vi "gaussian.vi"() -> ()   [LabVIEW 2015]
panel:
  out "Intensity Chart":dbl[][](graph)
  out "Waveform Chart":dbl[](graph)
  out "size(s)":i32
  in  "sigma":dbl(slide)=0.5 scale=-5.0..5.0
  in  "kernelSize":enum16{"3x3", "5x5", "7x7"}(ring)
  out "G":dbl[][](array[numeric])
  in  "dX":dbl=1.0 format="%#_13g"
  in  "sigma":dbl=0.8493
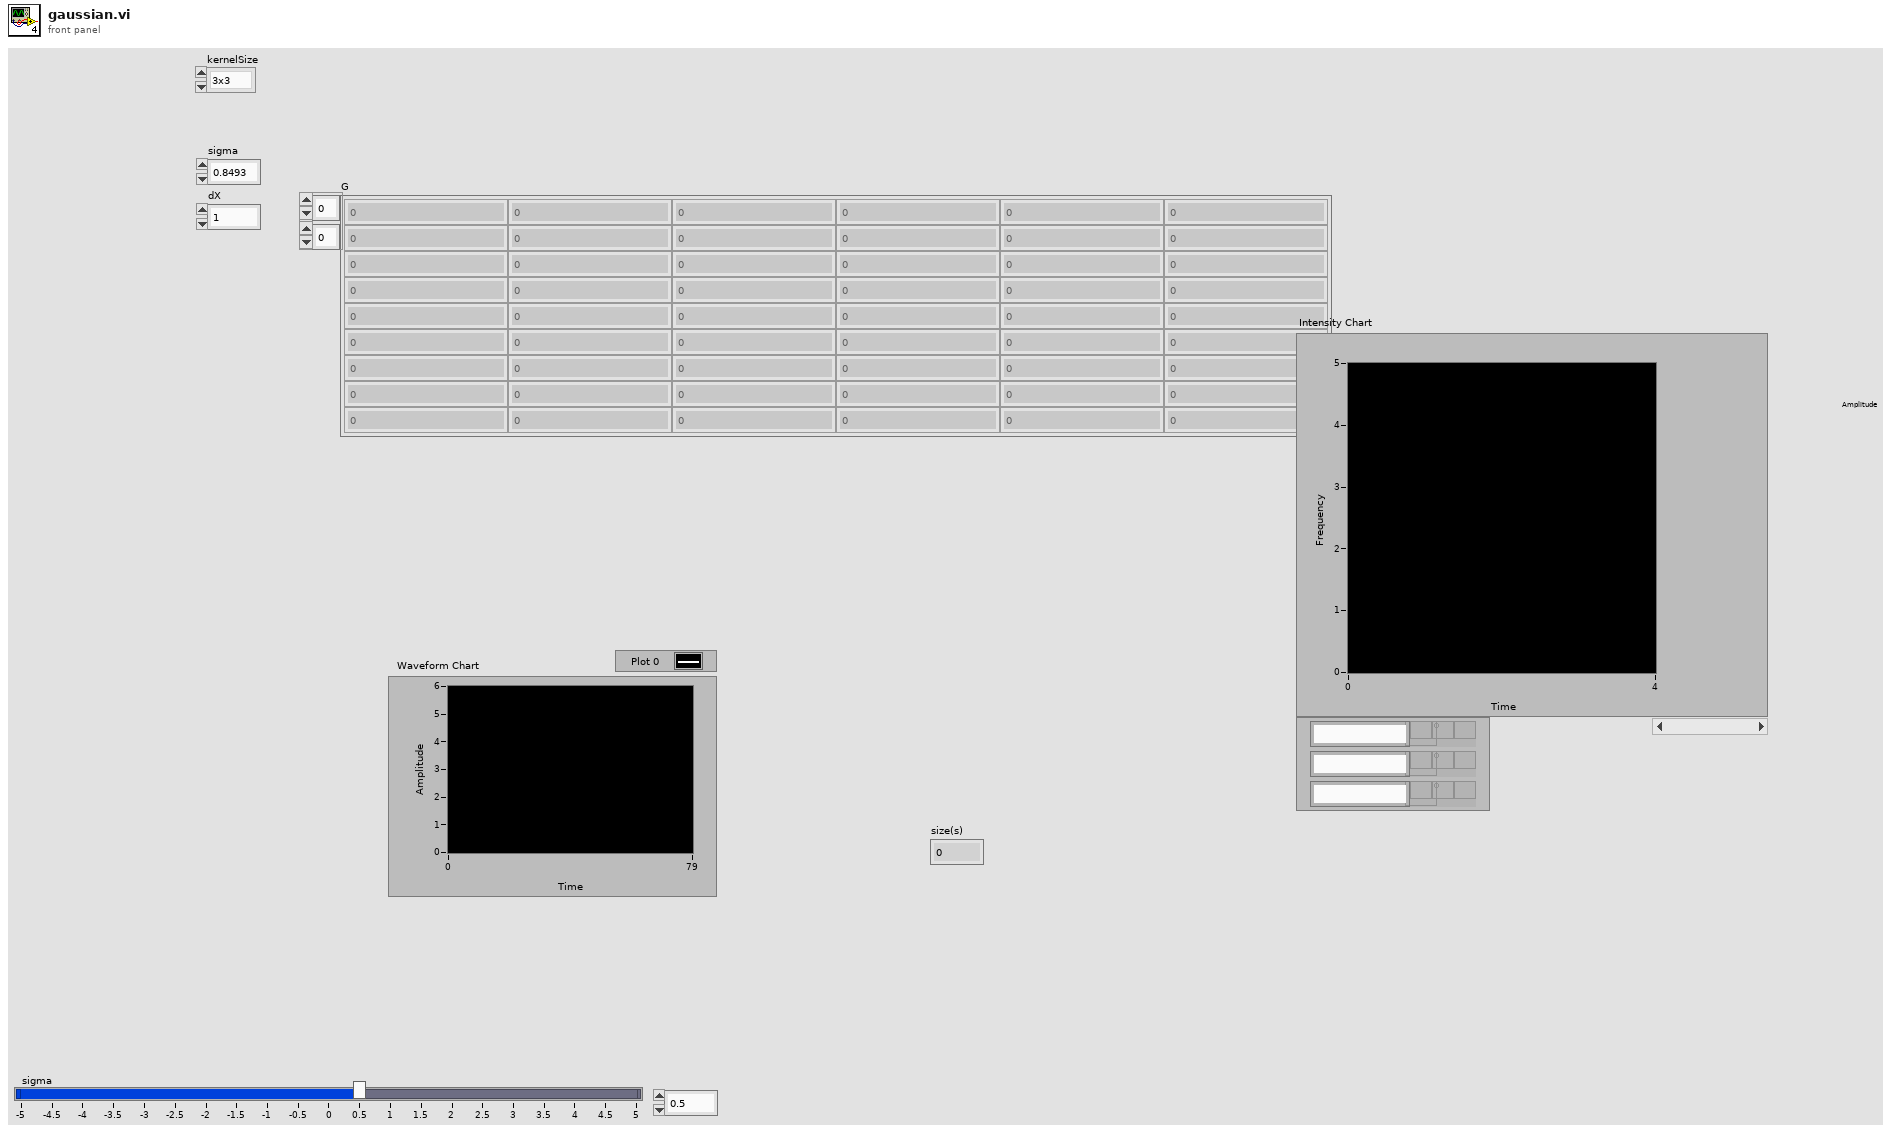
[diagram p1: front panel]
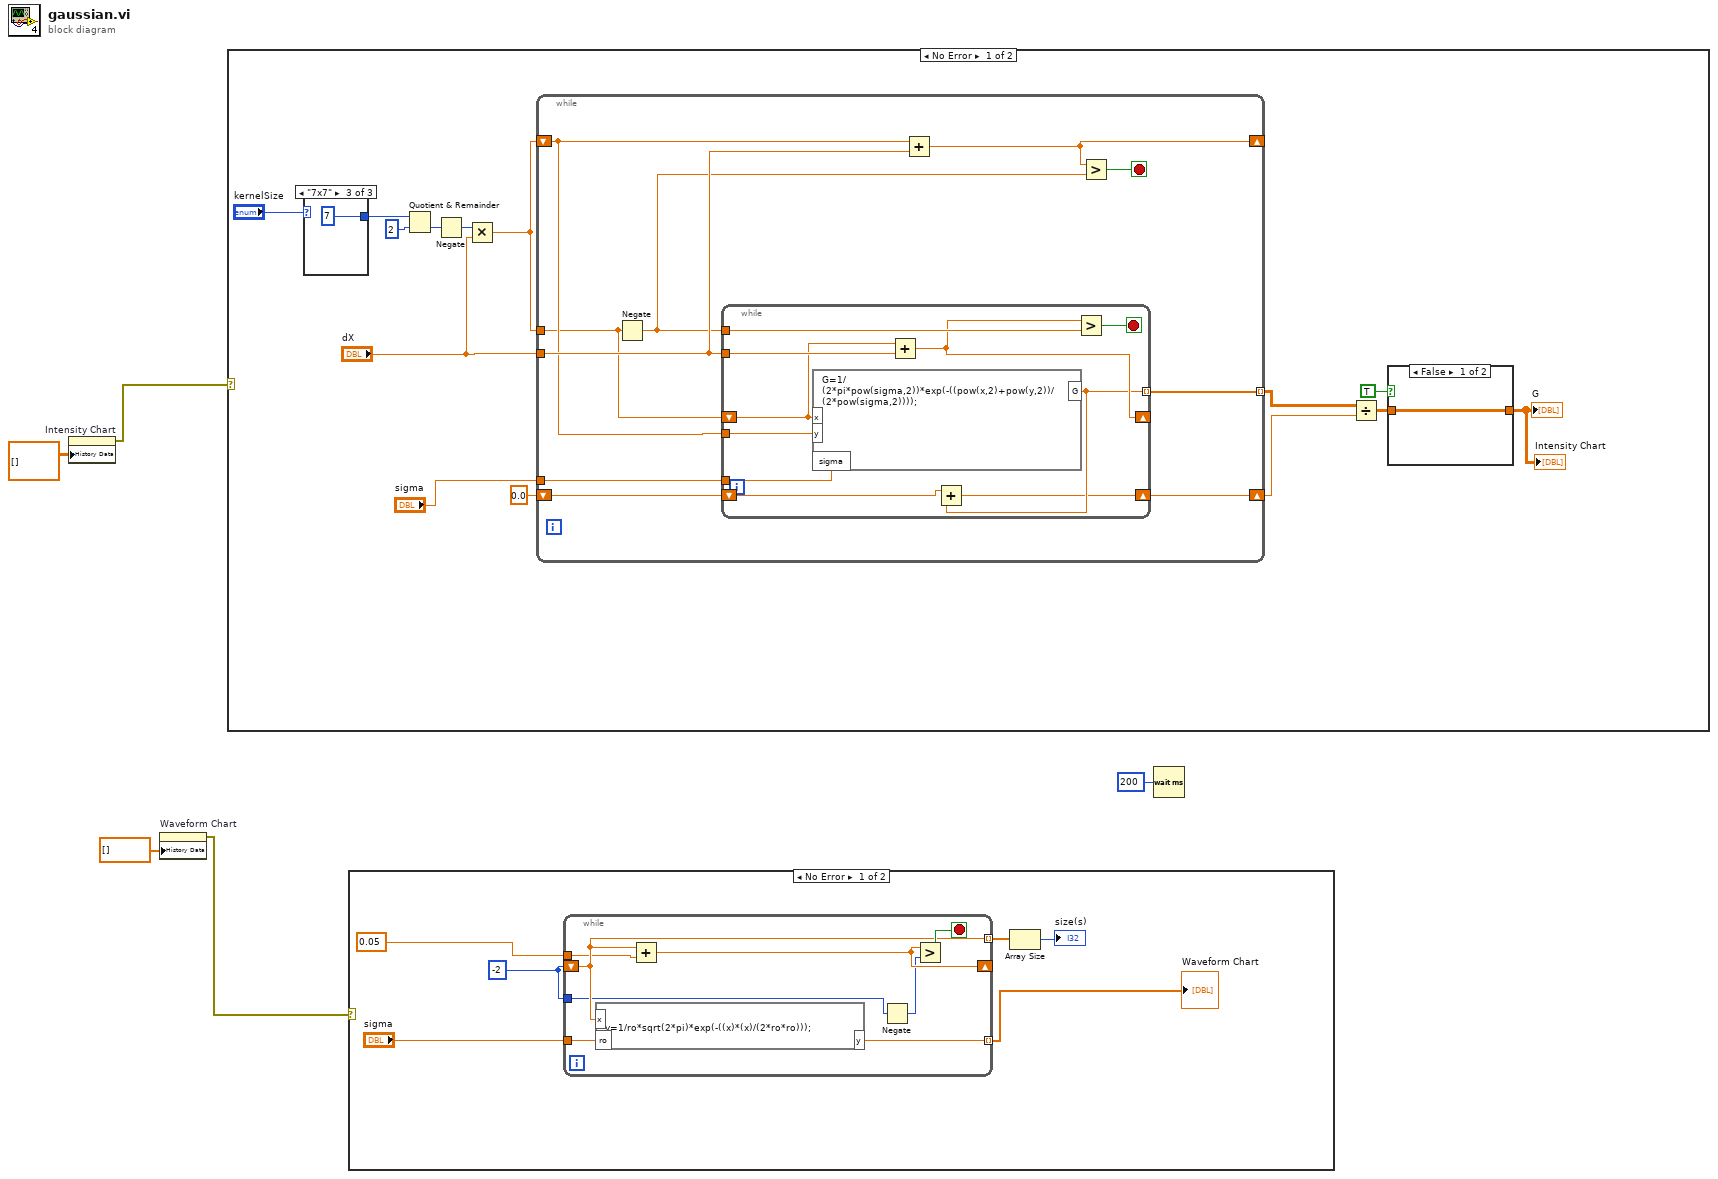
[diagram p0: block diagram]
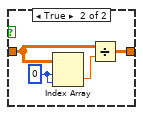
[diagram p2: hidden frame]
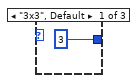
[diagram p3: hidden frame]
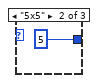
[diagram p4: hidden frame]
diagram:
  n1 = property on="Intensity Chart" class="IntChart (strict)"("History Data"=dbl[][] []) -> (error out=w2:errorcluster)  [unwired: 2 in, 1 out]
  n2 = property on="Waveform Chart" class="WFChart (strict)"("History Data"=dbl[] []) -> (error out=w4:errorcluster)  [unwired: 2 in, 1 out]
  n3 = case shown="No Error" w2 {
    frame No Error {
      n4 = case shown="\"7x7\"" "kernelSize" {
        tunnel: [3 5 7] -> w13
        frame "3x3", Default {
        }
        frame "5x5" {
        }
        frame "7x7" {
        }
      }
      n5 = Quotient & Remainder(x=w13, y=2) -> (floor(x/y)=w10:i32)  [unwired: 1 out]
      n6 = Negate(x=w10) -> (-x=w12:i32)
      n7 = Multiply(x=w12, y="dX") -> (x*y=w11:dbl)
      n8 = while {
        shift-right: [w32] -> _
        shift-left: w11 -> [w31]
        tunnel: "sigma" -> [w37]
        tunnel: [w36] -> w9 mode=indexing
        tunnel: "dX" -> [w35]
        tunnel: w11 -> [w30]
        shift-right: [w28] -> w18
        shift-left: 0.0 -> [w29]
        stop <- w34 stop-if-true
        n9 = Negate(x=w30) -> (-x=w33:dbl)
        n10 = while {
          tunnel: w37 -> [w47]
          tunnel: [w39] -> w36 mode=indexing
          tunnel: w35 -> [w46]
          tunnel: w33 -> [w44]
          tunnel: w31 -> [w43]
          shift-right: [w41] -> _
          shift-left: w30 -> [w42]
          shift-right: [w38] -> w28
          shift-left: w29 -> [w40]
          stop <- w45 stop-if-true
          n11 = formula code="G=1/(2*pi*pow(sigma,2))*exp(-((pow(x,2)+pow(y,2))/(2*pow(sigma,2))));"("x"=w42, "sigma"=w47, "y"=w43) -> ("G"=w39:dbl)
          n12 = Add(x=w42, y=w46) -> (x+y=w41:dbl)
          n13 = Add(x=w40, y=w39) -> (x+y=w38:dbl)
          n14 = Greater?(x=w41, y=w44) -> (0:w45:bool)
        }
        n15 = Add(x=w31, y=w35) -> (x+y=w32:dbl)
        n16 = Greater?(x=w32, y=w33) -> (0:w34:bool)
      }
      n17 = Divide(x=w9, y=w18) -> (x/y=w8:dbl[][])
      n18 = case shown="False" TRUE {
        tunnel: w8 -> [w20 w24]
        tunnel: [w20 w21] -> w7
        frame False {
        }
        frame True {
          w23 = 0 ("index (row)")
          n19 = Index Array(array=w24, index (row)=w23, index (col)=w23) -> (element=w22:dbl)
          n20 = Divide(x=w24, y=w22) -> (x/y=w21:dbl[][])
        }
      }
      "G" <- w7
      "Intensity Chart" <- w7
    }
    frame Error {
    }
  }
  n21 = case shown="No Error" w4 {
    frame No Error {
      w50 = -2
      n22 = while {
        shift-right: [w57] -> _
        shift-left: w50 -> [w58]
        tunnel: [w60] -> w48 mode=indexing
        tunnel: "sigma" -> [w59]
        tunnel: [w58] -> w52 mode=indexing
        tunnel: w50 -> [w55]
        tunnel: 0.05 -> [w56]
        stop <- w61 stop-if-true
        n23 = formula code="y=1/ro*sqrt(2*pi)*exp(-((x)*(x)/(2*ro*ro)));"("x"=w58, "ro"=w59) -> ("y"=w60:dbl)
        n24 = Add(x=w58, y=w56) -> (x+y=w57:dbl)
        n25 = Negate(x=w55) -> (-x=w54:i32)
        n26 = Greater?(x=w57, y=w54) -> (0:w61:bool)
      }
      "Waveform Chart" <- w48
      n27 = Array Size(array=w52) -> (size(s)=→"size(s)":i32)
    }
    frame Error {
    }
  }
  n28 = Wait (ms)(milliseconds to wait=u32 200) -> ()  [unwired: 1 out]
